vi "Read_Feedback_MsgQ.vi"(6 "timeout in ms (2000)":i32=2000, 8 "error in (no error)":errorcluster, 10 "ResponseAddr in":string="notif1") -> (0 "error out":errorcluster, 1 "timed out?":bool, 2 "Code":dbl, 3 "Data out":string[](array[string]))   [LabVIEW 2019, in "MsgQ.lvlib"]
uses:
  MsgQ.lvlib
  mmw_Service/TypeDef/NotifierQ.ctl
  mmw_Service/Service.lvlib
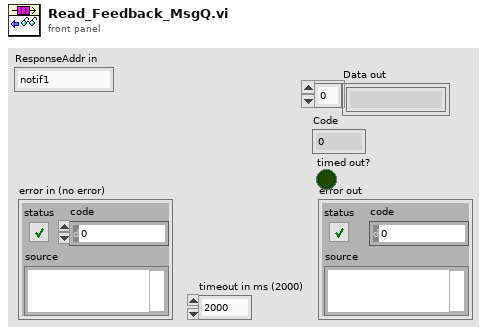
[diagram p1: front panel]
types:
  T1 = typedef "Service.lvlib/NotifierQ.ctl" = cluster{"Data":variant, "Code":dbl}
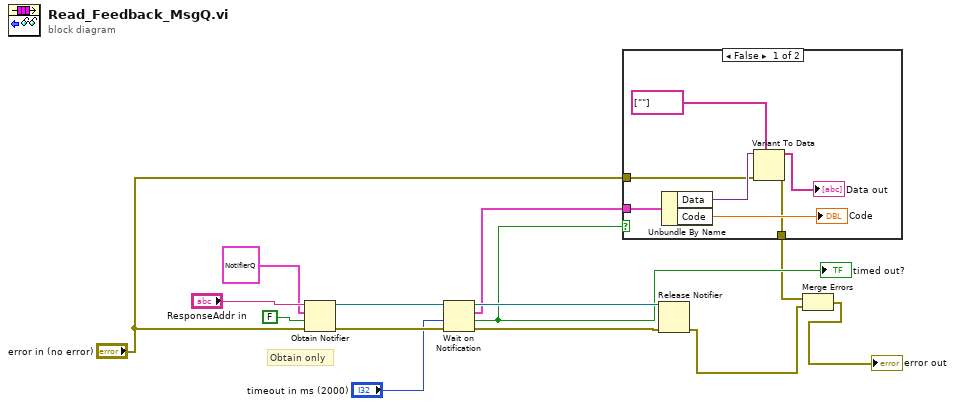
[diagram p0: block diagram]
diagram:
  # "Obtain only"
  n1 = Obtain Notifier(name (unnamed)="ResponseAddr in", notification data type=T1 {"Data"=variant(enum16{""} enum.""), "Code"=0.0}, create if not found? (T)=FALSE, error in (no error)="error in (no error)") -> (notifier out=w9:refnum<notifier>, error out=w11:errorcluster)  [unwired: 1 out]
  n2 = Wait on Notification(notifier=w9, timeout in ms (-1)="timeout in ms (2000)", error in (no error)=w11) -> (notifier out=w12:refnum<notifier>, notification=w6:T1, timed out?=w5:bool, error out=w10:errorcluster)  [unwired: 1 in]
  "timed out?" <- w5
  n3 = case shown="False" w5 {
    tunnel: w6 -> [w21 _]
    tunnel: "error in (no error)" -> [w16 w22]
    tunnel: [w15 w22] -> w3
    frame False {
      n4 = Unbundle By Name(w21) -> ("Data"=w19:variant, "Code"=→"Code":dbl)
      n5 = Variant To Data(error in=w16, type=string[] [""] ("Data in 2"), Variant=w19) -> (data=→"Data out":string[], error out=w15:errorcluster)
    }
    frame True {
    }
  }
  n6 = Release Notifier(notifier=w12, error in (no error)=w10) -> (error out=w2:errorcluster)  [unwired: 1 in, 2 out]
  n7 = Merge Errors(w3, w2) -> (→"error out":errorcluster)
